vi "Init.vi"(8 "error in (no error)":errorcluster, 11 "Status Request":refnum<user-event>) -> (0 "error out":errorcluster, 3 "TimerStatusController out":refnum<class "TimerStatusController.lvclass">)   [LabVIEW 2020, in "Timer Demo.lvlib" / "TimerStatusController.lvclass"]
uses:
  TimerStatusController.lvclass
  Timer Status Response.ctl
  Timer Demo.lvlib
  Timer Status Request.ctl
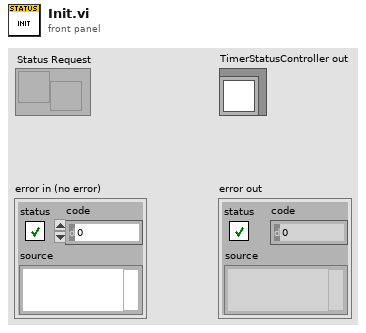
[diagram p1: front panel]
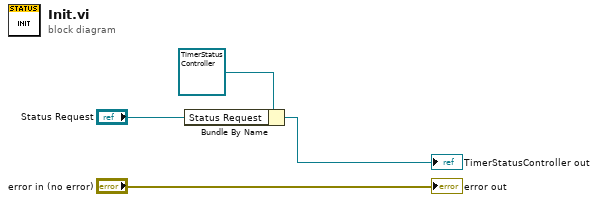
[diagram p0: block diagram]
diagram:
  n1 = Bundle By Name(cluster=refnum<class "TimerStatusController.lvclass"> refnum ("TimerStatusController in"), "Status Request"="Status Request") -> (→"TimerStatusController out":refnum<class "TimerStatusController.lvclass">)
  "error out" <- "error in (no error)"
